vi "ANDO tracedownload_2011 version.vi"() -> ()   [LabVIEW 2011]
uses:
  <vilib>/Utility/file.llb/Write To Spreadsheet File (DBL).vi
panel:
  in  "export graph path":path=path "C:/Users/VGroup/Desktop/data/20140419/111"
  out "XY Graph":cluster{"Wavelength":sgl[], "Level":sgl[]}(graph)
  in  "Save data?":bool=TRUE
  out "Error Out":errorcluster
  in  "Error In":errorcluster
  in  "Trace (0:A)":enum16{"A", "B", "C"}(ring)
  in  "VISA session":refnum<visa-resource-name>="GPIB0::1::INSTR"
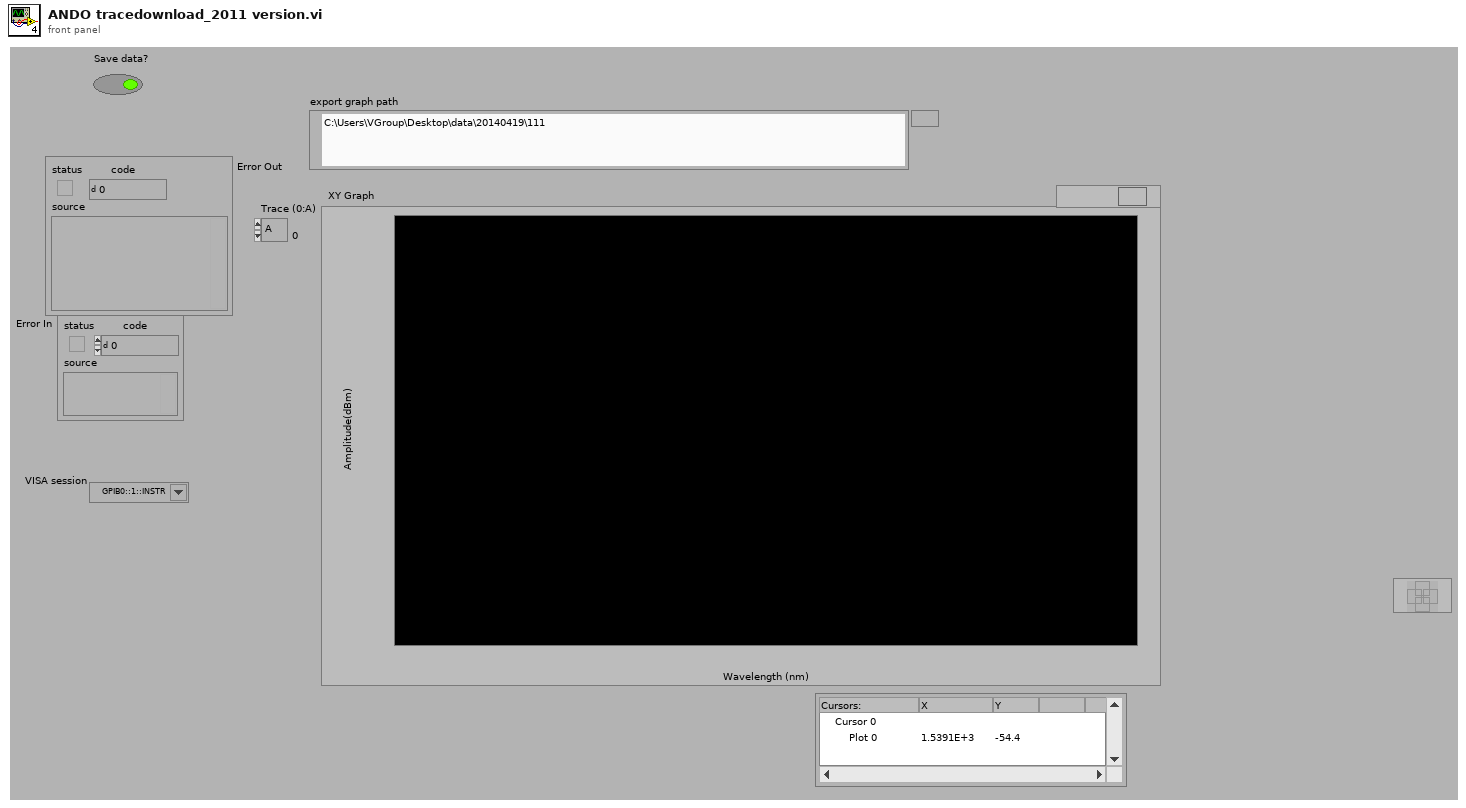
[diagram p1: front panel]
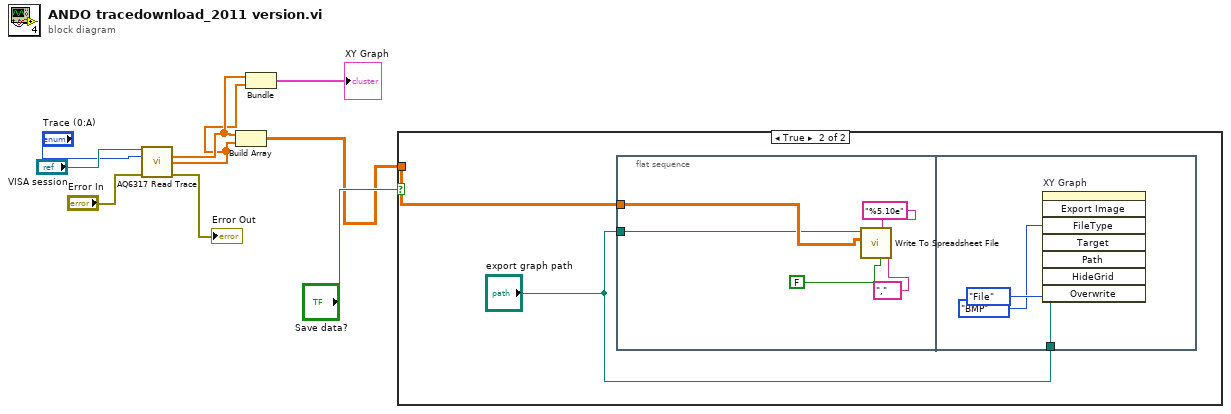
[diagram p0: block diagram]
diagram:
  n1 = call <instrlib>:"AQ6317 Read Trace.vi"("VISA session"="VISA session", "Trace (0:A)"="Trace (0:A)", "Error In"="Error In") -> ("Wavelength"=w3:sgl[], "Level"=w2:sgl[], "Error Out"=→"Error Out":errorcluster)  [unwired: 7 in, 3 out]
  n2 = Build Array(w3, w2) -> (w4:sgl[][])
  n3 = Bundle("Wavelength"=w3, "Level"=w2) -> (→"XY Graph":cluster{"Wavelength":sgl[], "Level":sgl[]})  [unwired: 1 in]
  n4 = case shown="True" "Save data?" {
    tunnel: w4 -> [_ w11]
    frame False {
    }
    frame True {
      n5 = flat-sequence {
        tunnel: w11 -> [w16]
        tunnel: "export graph path" -> [w12]
        tunnel: "export graph path" -> [w17]
        frame #0 {
          n6 = call-poly <vilib>:"Write To Spreadsheet File.vi"("delimiter (\\t)"="," ("delimiter (Tab)"), "transpose? (no:F)"=FALSE, "format (%.3f)"="%5.10e", "2D data"=w16, "file path (dialog if empty)"=w12) -> ()  [unwired: 3 in, 1 out]
        }
        frame #1 {
          n7 = invoke on="XY Graph" class="XYGraph (strict)" method="Export Image"("FileType"=enum32{"BMP", "EPS", "EMF", "PICT"}."BMP" ("File Type"), "Target"=enum32{"File", "Clipboard"}."File", "Path"=w17) -> ()  [unwired: 5 in, 8 out]
        }
      }
    }
  }
